vi "CreateExperiments.vi"(0 "object in":refnum<class "ExperimentSeries2.lvclass">, 1 "SeriesPath":path, 2 "Analog Discovery Settings":T2, 3 "Dyamic Camera Start Time":bool, 4 "GlobalExposure":bool, 5 "error in (no error)":errorcluster, 6 "Frequency List":dbl[](array[numeric])=[0.0, 1.0], 7 "Frames":i32, 8 "Repeats":i32, 9 "ExposureTime(ms)":dbl, 10 "Dynamic Frequency":bool, 11 "Flush Settings":T1, 13 "Camera Start Array(s)":dbl[](array[numeric])) -> (14 "object out":refnum<class "ExperimentSeries2.lvclass">, 16 "Array":refnum<class "Experiment2.lvclass">[](array[class]), 19 "error out":errorcluster)   [LabVIEW 2024, in "ExperimentSeries2.lvclass"]
uses:
  ExperimentSeries2.lvclass
  Experiment2_class/Experiment2.lvclass
  AD2_DO_SDK_class/DOTrigger.ctl
  AD2_WFG_SDK_class/AD2TriggerSources.ctl
  AD2_WFG_SDK_class/WFG.ctl
  AD2_WFG_SDK_class/WFGCh.ctl
  ExperimentSeries2.lvclass/ExperimentSeries2.ctl
  AD2_SDK_class/AD2_SDK.lvclass
  AD2_DO_SDK_class/AD2_DO_SDK.lvclass
  AD2_WFG_SDK_class/AD2_WFG_SDK.lvclass
panel:
  # "0 init\n1 low\n2 high\n3 tristate"
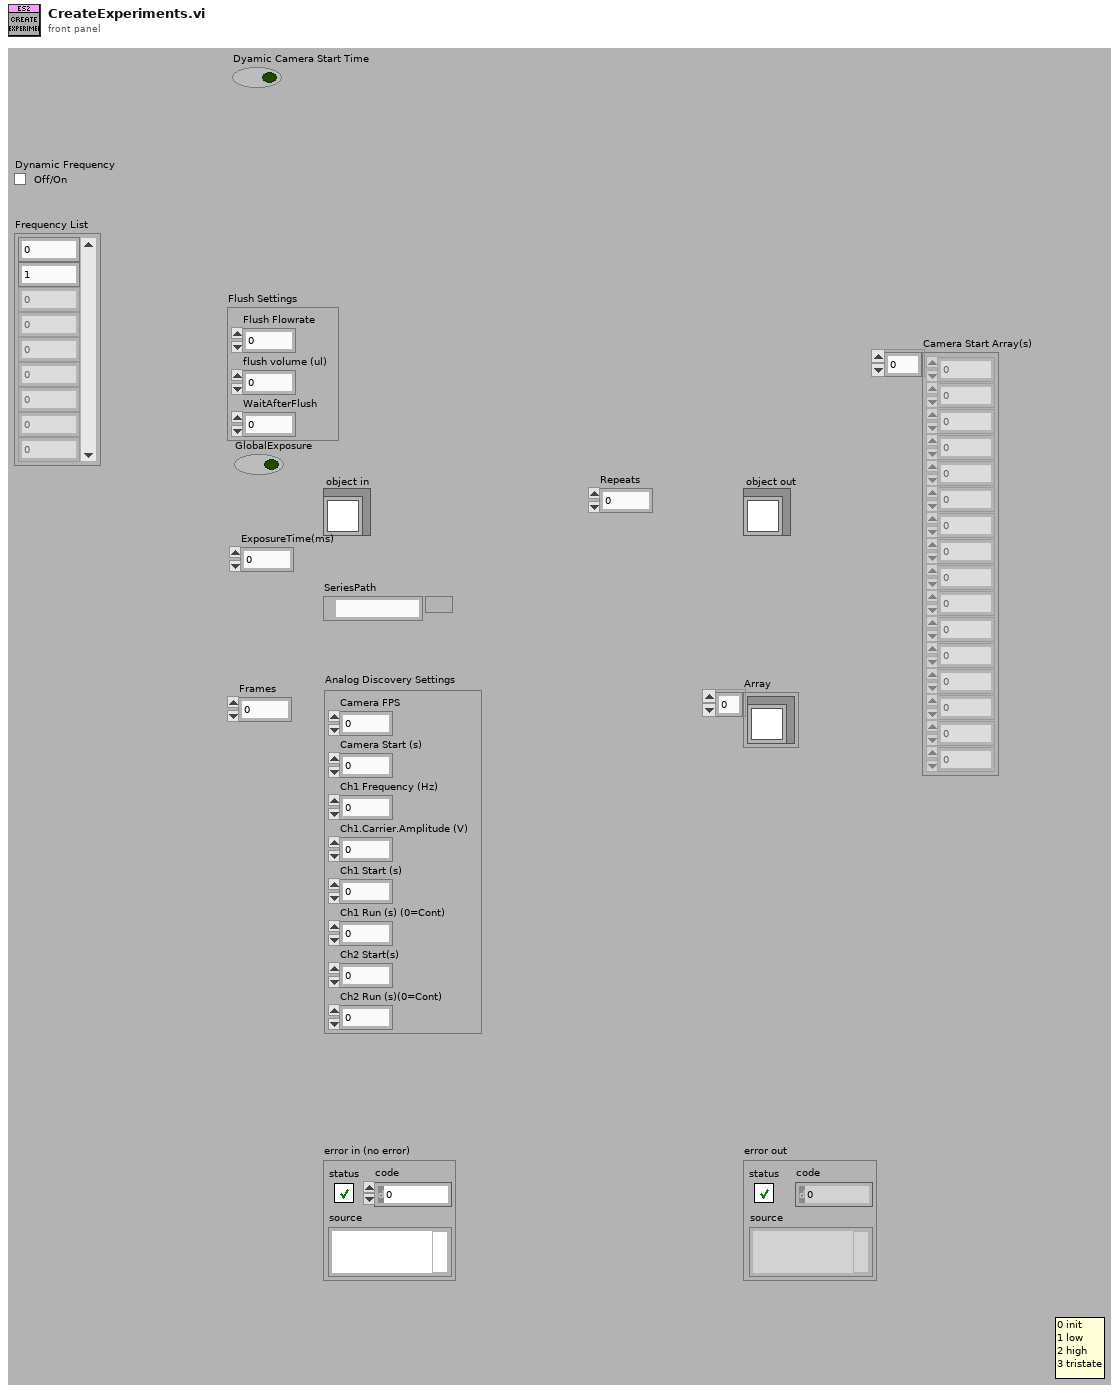
[diagram p1: front panel]
types:
  T1 = cluster{"Flush Flowrate":dbl, "flush volume (ul)":dbl, "WaitAfterFlush":dbl}
  T2 = cluster{"Camera FPS":dbl, "Camera Start (s)":dbl, "Ch1 Frequency (Hz)":dbl, "Ch1.Carrier.Amplitude (V)":dbl, "Ch1 Start (s)":dbl, "Ch1 Run (s) (0=Cont)":dbl, "Ch2 Start(s)":dbl, "Ch2 Run (s)(0=Cont)":dbl}
  T3 = cluster{"Master Pulse Settings":cluster{"Mode":u32, "Source":u32, "Interval":dbl, "Burst":u32}, "Capture mode":i32, "Frames":i32, "Dcam Trigger Source":i32, "External Options":cluster{"Polarity":i32, "Delay":dbl}, "ExposureTime(ms)":dbl}
  T4 = typedef "AD2_WFG_SDK.lvclass/WFG.ctl" = cluster{"Running":bool, "Ch1":T5, "Ch2":T5, "SyncronizeState":enum16{"Independent", "Ch1Master", "Ch2Master"}}
  T5 = typedef "AD2_WFG_SDK.lvclass/WFGCh.ctl" = cluster{"idxChannel":i32, "Settings out of range":bool, "Carrier":cluster{"Frequency (Hz)":dbl, "Amplitude (V)":dbl, "Offset(V)":dbl, "Symmetry(%) ":dbl, "Phase(Deg)":dbl, "Function":u16, "Enable":bool}, "Trigger":cluster{"secRun(0=Cont)":dbl, "secWait":dbl, "cRepeat(0=inf)":i32, "Repeat Trigger":bool, "TrigrSrc":T6}, "FM Mod":cluster{"Frequency (Hz)":dbl, "Amplitude (%)":dbl, "Offset(V)":dbl, "Symmetry(%) ":dbl, "Phase(Deg)":dbl, "Function 2":u16, "Enable":bool}}
  T6 = typedef "AD2_SDK.lvclass/AD2TriggerSources.ctl" = enum8{"trigrsrcNone", "trigsrcPC", "trigsrcDetectorAnalogIn", "trigsrcDetectorDigitalIn", "trigsrcAnalogIn", "trigsrcDigitalIn", "trigsrcDigitalOut", "trigsrcAnalogOut1", "trigsrcAnalogOut2", "trigsrcAnalogOut3", "trigsrcAnalogOut4", "trigsrcExternal1", "trigsrcExternal2", "trigsrcExternal3", "trigsrcExternal4", ""}
  T7 = typedef "AD2_DO_SDK.lvclass/DOTrigger.ctl" = cluster{"secRun(0=Cont)":dbl, "secWait":dbl, "cRepeat(0=inf)":i32, "Repeat Trigger":bool, "TrigrSrc":T6}
  T8 = cluster{"DO Trigger":T7, "ClockSettings":cluster{"Frequency":dbl, "Enable":bool, "IdleState":enum16{"Initial", "Low", "High", "Z"}}[]}
  T9 = cluster{"Frequency":dbl, "Enable":bool, "IdleState":enum16{"Initial", "Low", "High", "Z"}}
  T10 = cluster{"Frequency":dbl, "Enable":bool, "IdleState":enum16{"Initial", "Low", "High", "Z"}}[]
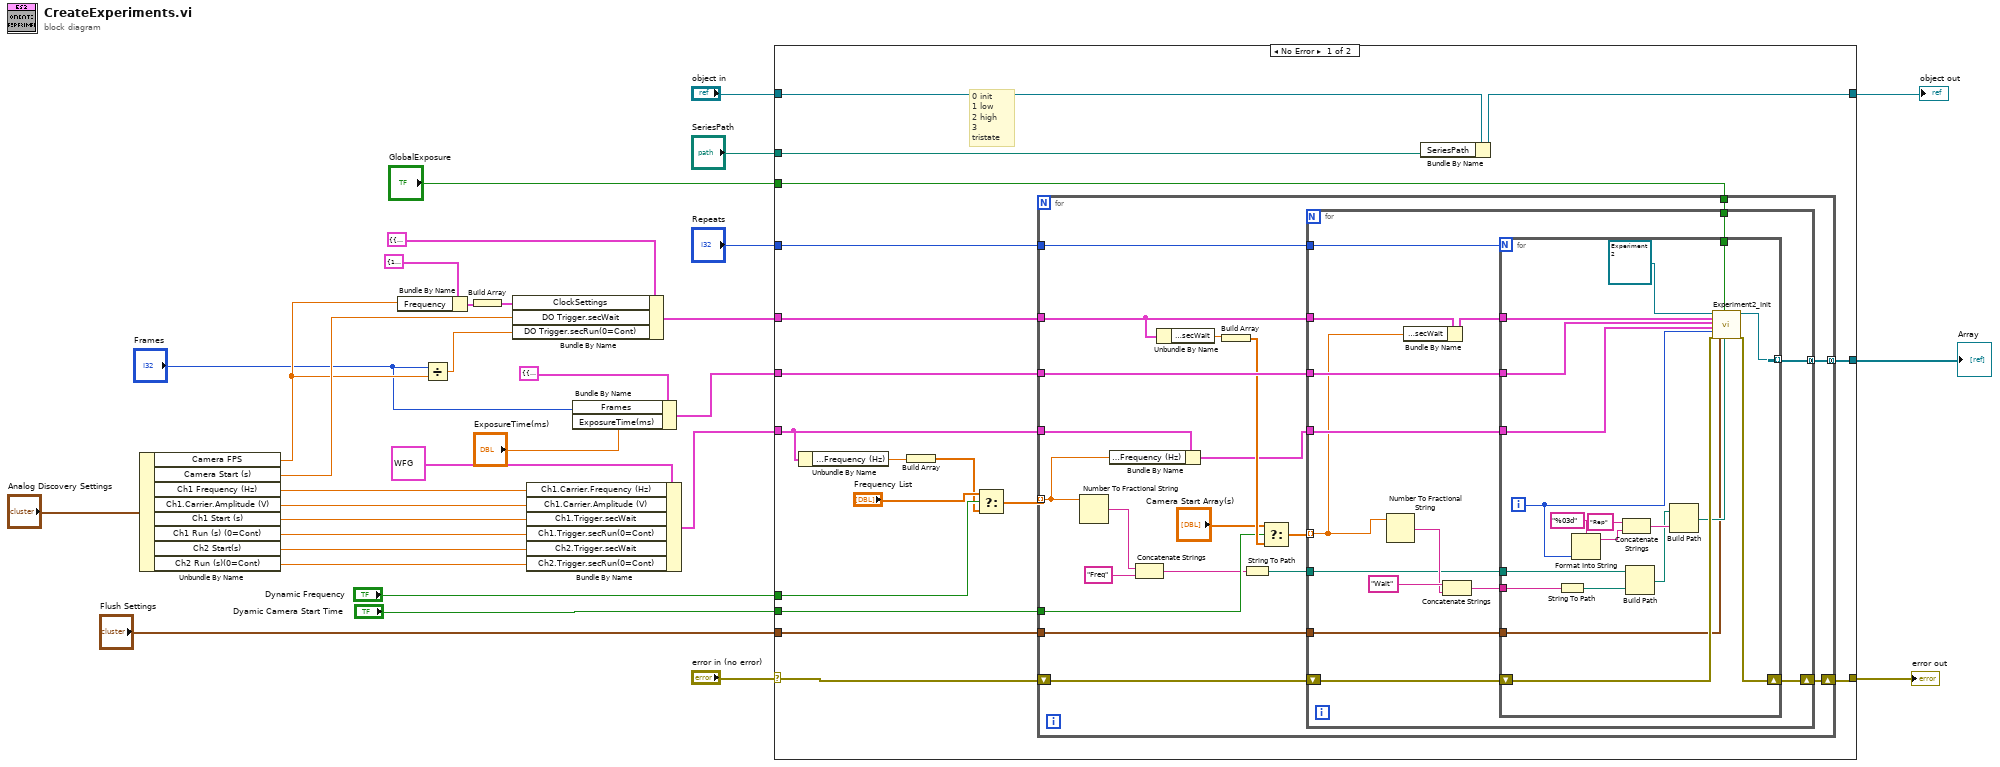
[diagram p0: block diagram]
diagram:
  n1 = Unbundle By Name("Analog Discovery Settings") -> ("Camera FPS"=w6:dbl, "Camera Start (s)"=w17:dbl, "Ch1 Frequency (Hz)"=w16:dbl, "Ch1.Carrier.Amplitude (V)"=w15:dbl, "Ch1 Start (s)"=w14:dbl, "Ch1 Run (s) (0=Cont)"=w13:dbl, "Ch2 Start(s)"=w12:dbl, "Ch2 Run (s)(0=Cont)"=w11:dbl)
  n2 = Bundle By Name(cluster=T9 {"Frequency"=100.0, "Enable"=TRUE, "IdleState"=enum."Low"} ("Clock Settings"), "Frequency"=w6) -> (w23:T9)
  n3 = Divide(x="Frames", y=w6) -> (x/y=w4:dbl)
  n4 = Build Array(w23) -> (w22:T10)
  n5 = Bundle By Name(cluster=T8 {"DO Trigger"={"secRun(0=Cont)"=2.0, "secWait"=0.0, "cRepeat(0=inf)"=1, "Repeat Trigger"=FALSE, "TrigrSrc"=enum."trigsrcPC"}, "ClockSettings"=[{"Frequency"=100.0, "Enable"=TRUE, "IdleState"=enum."Low"}]} ("DOClockSettings 2"), "ClockSettings"=w22, "DO Trigger.secWait"=w17, "DO Trigger.secRun(0=Cont)"=w4) -> (w21:T8)
  n6 = Bundle By Name(cluster=T4 {"Running"=TRUE, "Ch1"={"idxChannel"=0, "Settings out of range"=FALSE, "Carrier"={"Frequency (Hz)"=10.0, "Amplitude (V)"=2.0, "Offset(V)"=0.0, "Symmetry(%) "=50.0, "Phase(Deg)"=0.0, "Function"=1, "Enable"=TRUE}, "Trigger"={"secRun(0=Cont)"=1.0, "secWait"=0.1, "cRepeat(0=inf)"=1, "Repeat Trigger"=FALSE, "TrigrSrc"=enum."trigsrcPC"}, "FM Mod"={"Frequency (Hz)"=1000.0, "Amplitude (%)"=1.0, "Offset(V)"=0.0, "Symmetry(%) "=50.0, "Phase(Deg)"=0.0, "Function 2"=1, "Enable"=FALSE}}, "Ch2"={"idxChannel"=1, "Settings out of range"=FALSE, "Carrier"={"Frequency (Hz)"=0.01, "Amplitude (V)"=5.0, "Offset(V)"=0.0, "Symmetry(%) "=50.0, "Phase(Deg)"=0.0, "Function"=2, "Enable"=TRUE}, "Trigger"={"secRun(0=Cont)"=1.0, "secWait"=0.0, "cRepeat(0=inf)"=1, "Repeat Trigger"=FALSE, "TrigrSrc"=enum."trigsrcPC"}, "FM Mod"={"Frequency (Hz)"=1000.0, "Amplitude (%)"=1.0, "Offset(V)"=0.0, "Symmetry(%) "=50.0, "Phase(Deg)"=0.0, "Function 2"=1, "Enable"=FALSE}}, "SyncronizeState"=enum."Independent"} ("WFGConfig"), "Ch1.Carrier.Frequency (Hz)"=w16, "Ch1.Carrier.Amplitude (V)"=w15, "Ch1.Trigger.secWait"=w14, "Ch1.Trigger.secRun(0=Cont)"=w13, "Ch2.Trigger.secWait"=w12, "Ch2.Trigger.secRun(0=Cont)"=w11) -> (w19:T4)
  n7 = Bundle By Name(cluster=T3 {"Master Pulse Settings"={"Mode"=1, "Source"=1, "Interval"=1.0, "Burst"=0}, "Capture mode"=1, "Frames"=0, "Dcam Trigger Source"=2, "External Options"={"Polarity"=2, "Delay"=0.0}, "ExposureTime(ms)"=0.0} ("Sequence Settings 2"), "Frames"="Frames", "ExposureTime(ms)"="ExposureTime(ms)") -> (w9:T3)
  n8 = case shown="No Error" "error in (no error)" {
    selector: "error in (no error)" -> [w48 w106]
    tunnel: [w47 w106] -> w31
    tunnel: [w49 w105] -> w29
    tunnel: "object in" -> [w50 w105]
    tunnel: [w46 _] -> w28
    tunnel: "SeriesPath" -> [w45 _]
    tunnel: w19 -> [w38 _]
    tunnel: w9 -> [w44 _]
    tunnel: w21 -> [w40 _]
    tunnel: "Repeats" -> [w43 _]
    tunnel: "Flush Settings" -> [w42 _]
    tunnel: "GlobalExposure" -> [w41 _]
    tunnel: "Dyamic Camera Start Time" -> [w39 _]
    tunnel: "Dynamic Frequency" -> [w34 _]
    frame No Error {
      # "0 init\n1 low\n2 high\n3 tristate"
      n9 = Unbundle By Name(w38) -> ("Ch1.Carrier.Frequency (Hz)"=w37:dbl)
      n10 = Build Array(w37) -> (w33:dbl[])
      n11 = Select(t="Frequency List", s=w34, f=w33) -> (s? t:f=w36:dbl[])
      n12 = for {
        tunnel: [w68] -> w46 mode=concatenating
        tunnel: w44 -> [w67]
        tunnel: w43 -> [w66]
        tunnel: w38 -> [w57]
        tunnel: w42 -> [w65]
        tunnel: w41 -> [w64]
        tunnel: w40 -> [w63]
        tunnel: w39 -> [w58]
        shift-right: [w69] -> w47
        shift-left: w48 -> [w70]
        tunnel: w36 -> [w55] mode=indexing
        n13 = Number To Fractional String(number=w55) -> (F-format string=w51:string)  [unwired: 3 in]
        n14 = Bundle By Name(cluster=w57, "Ch1.Carrier.Frequency (Hz)"=w55) -> (w56:T4)
        n15 = Concatenate Strings(w51, "Freq" ("string")) -> (w53:string)
        n16 = Unbundle By Name(w63) -> ("DO Trigger.secWait"=w62:dbl)
        n17 = Build Array(w62) -> (w61:dbl[])
        n18 = String To Path(string=w53) -> (path=w52:path)
        n19 = Select(t="Camera Start Array(s)", s=w58, f=w61) -> (s? t:f=w59:dbl[])
        n20 = for {
          tunnel: [w83] -> w68 mode=concatenating
          tunnel: w67 -> [w82]
          tunnel: w63 -> [w81]
          tunnel: w66 -> [w80]
          tunnel: w56 -> [w77]
          tunnel: w65 -> [w79]
          tunnel: w64 -> [w78]
          shift-right: [w84] -> w69
          shift-left: w70 -> [w85]
          tunnel: w59 -> [w73] mode=indexing
          tunnel: w52 -> [w71]
          n21 = Number To Fractional String(number=w73) -> (F-format string=w74:string)  [unwired: 3 in]
          n22 = Bundle By Name(cluster=w81, "DO Trigger.secWait"=w73) -> (w76:T8)
          n23 = Concatenate Strings("Wait" ("string"), w74) -> (w72:string)
          n24 = for {
            N: w80 -> [_]
            shift-right: [w101] -> w84
            shift-left: w85 -> [w103]
            tunnel: [w102] -> w83 mode=indexing
            tunnel: w76 -> [w94]
            tunnel: w82 -> [w93]
            tunnel: w77 -> [w92]
            tunnel: w79 -> [w91]
            tunnel: w78 -> [w90]
            tunnel: w72 -> [w89]
            tunnel: w71 -> [w86]
            i -> [w99]
            n25 = String To Path(string=w89) -> (path=w88:path)
            n26 = Format Into String(format string="%03d", w99) -> (resulting string=w98:string)  [unwired: 2 in, 1 out]
            n27 = Concatenate Strings("Rep" ("string"), w98) -> (w96:string)
            n28 = Build Path(base path=w86, name or relative path=w88) -> (appended path=w87:path)
            n29 = Build Path(base path=w87, name or relative path=w96) -> (appended path=w95:path)
            n30 = call "Experiment2_Init.vi"("object in"=refnum<class "Experiment2.lvclass"> refnum, "DOClockSettings"=w94, "Sequence Settings"=w93, "WFGConfig"=w92, "Repeat ID"=w99, "error in (no error)"=w103, "Flush Settings"=w91, "GlobalExposure"=w90, "ExperimentFolder"=w95) -> ("object out"=w102:refnum<class "Experiment2.lvclass">, "error out"=w101:errorcluster)  [unwired: 9 in]
          }
        }
      }
      n31 = Bundle By Name(cluster=w50, "SeriesPath"=w45) -> (w49:refnum<class "ExperimentSeries2.lvclass">)
    }
    frame Error {
    }
  }
  "error out" <- w31
  "object out" <- w29
  "Array" <- w28
